vi "RESET_SENSOR.vi"(10 "argv":string[](array[string]), 11 "args":u8) -> ()   [LabVIEW 2011]
panel:
  in  "Array":T1(array[cluster])=[{"name"="gyro_pitch", "sensor"=enum."pitch_gyro"}, {"name"="gyro_yaw", "sensor"=enum."yaw_gyro"}, {"name"="drive_encoders", "sensor"=enum."drive_encoders"}]
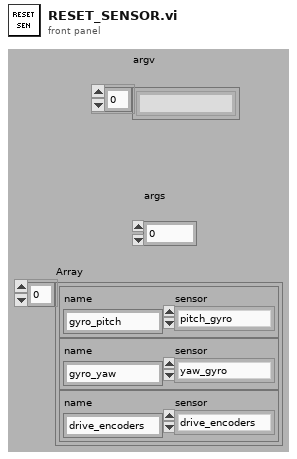
[diagram p1: front panel]
types:
  T1 = cluster{"name":string, "sensor":enum16{"pitch_gyro", "yaw_gyro", "drive_encoders"}}[]
  T2 = enum16{"pitch_gyro", "yaw_gyro", "drive_encoders"}
  T3 = typedef "WPI_GyroDevRef.ctl" = cluster{"DevStatus":errorcluster, "Analog Module":T4, "Analog Channel":T5, "Offset":dbl, "Gain (VoltsPerDegree/Second)":dbl}
  T4 = typedef "FPGA_TypedefAnalogModule.ctl" = enum16{"Analog Module 1", "Analog Module 2"}
  T5 = typedef "FPGA_AIChannel.ctl" = enum8{"AI 1", "AI 2", "AI 3", "AI 4", "AI 5", "AI 6", "AI 7", "AI 8", "Invalid"}
  T6 = typedef "WPI_EncoderDevRef.ctl" = cluster{"DevStatus":errorcluster, "EncoderIndex":T7, "CounterIndex":T8, "DistancePerCount":dbl, "Decoding Type":T9}
  T7 = typedef "FPGA_EncoderIdx.ctl" = enum8{"Enc 0", "Enc 1", "Enc 2", "Enc 3", "Invalid"}
  T8 = typedef "FPGA_CounterCtrSystemIndex.ctl" = enum8{"Ctr 0", "Ctr 1", "Ctr 2", "Ctr 3", "Ctr 4", "Ctr 5", "Ctr 6", "Ctr 7", "Invalid"}
  T9 = typedef "WPI_EncoderType.ctl" = enum16{"1x", "2x", "4x"}
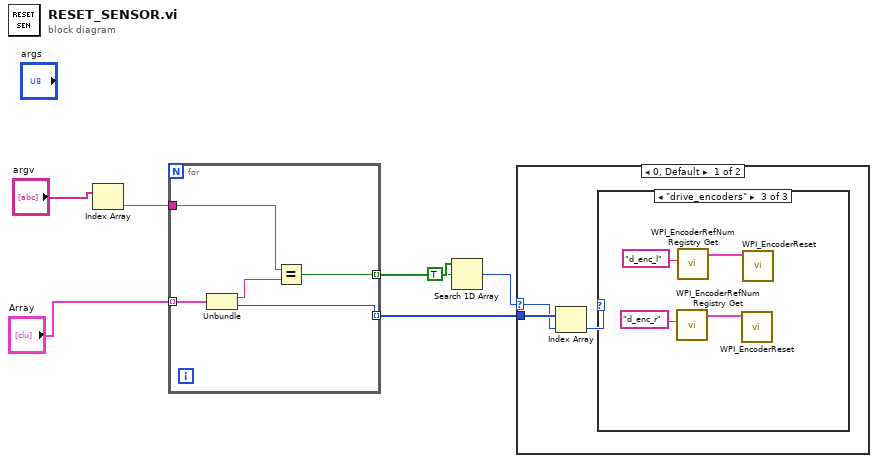
[diagram p0: block diagram]
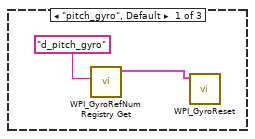
[diagram p2: hidden frame]
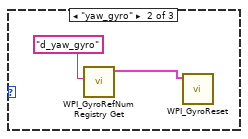
[diagram p3: hidden frame]
diagram:
  n1 = Index Array(array="argv") -> (element=w5:string)  [unwired: 1 in]
  n2 = for {
    tunnel: "Array" -> [w12] mode=indexing
    tunnel: w5 -> [w10]
    tunnel: [w9] -> w4 mode=indexing
    tunnel: [w8] -> w1 mode=indexing
    n3 = Unbundle(w12) -> ("name"=w11:string, "sensor"=w8:T2)
    n4 = Equal?(x=w10, y=w11) -> (x = y?=w9:bool)
  }
  n5 = Search 1D Array(1D array=w4, element=TRUE) -> (index of element=w2:i32)  [unwired: 1 in]
  n6 = case shown="0, Default" w2 {
    selector: w2 -> [w14 _]
    tunnel: w1 -> [w15 _]
    frame 0, Default {
      n7 = Index Array(array=w15, index=w14) -> (element=w13:T2)
      n8 = case shown="\"drive_encoders\"" w13 {
        frame "pitch_gyro", Default {
          n9 = call <vilib>:"WPI_GyroRefNum Registry Get.vi"("refnum name"="d_pitch_gyro") -> ("GyroDevRef"=w16:T3)  [unwired: 9 in, 1 out]
          n10 = call <vilib>:"WPI_GyroReset.vi"("GyroDevRef"=w16) -> ()  [unwired: 9 in, 2 out]
        }
        frame "yaw_gyro" {
          n11 = call <vilib>:"WPI_GyroRefNum Registry Get.vi"("refnum name"="d_yaw_gyro") -> ("GyroDevRef"=w18:T3)  [unwired: 9 in, 1 out]
          n12 = call <vilib>:"WPI_GyroReset.vi"("GyroDevRef"=w18) -> ()  [unwired: 9 in, 2 out]
        }
        frame "drive_encoders" {
          n13 = call <vilib>:"WPI_EncoderRefNum Registry Get.vi"("refnum name"="d_enc_r") -> ("EncoderDevRef"=w20:T6)  [unwired: 9 in, 1 out]
          n14 = call <vilib>:"WPI_EncoderRefNum Registry Get.vi"("refnum name"="d_enc_l") -> ("EncoderDevRef"=w22:T6)  [unwired: 9 in, 1 out]
          n15 = call <vilib>:"WPI_EncoderReset.vi"("EncoderDevRef"=w20) -> ()  [unwired: 9 in, 2 out]
          n16 = call <vilib>:"WPI_EncoderReset.vi"("EncoderDevRef"=w22) -> ()  [unwired: 9 in, 2 out]
        }
      }
    }
    frame -1 {
    }
  }
